vi "逐點分段offset改善、比較 2.vi"() -> ()   [LabVIEW 2017]
uses:
  <vilib>/Utility/miscctls.llb/LVPointDoubleTypeDef.ctl
panel:
  out "size(s)":i32
  out "Voltgae":dbl[](array[numeric])
  out "Voltage Position":cluster{"Speed":dbl[], "Position":dbl[]}(graph)
  out "element":T1
  in  "file path (use dialog)":path
  out "X  Position":dbl=1500.0
  out "max index(es)":i32=900
  out "Y max spped":dbl=50000.0
  out "NO OFFSET Graph":cluster{"Speed":dbl[], "Position":dbl[]}(graph)
  in  "OFFSET":dbl=0.6 format="%#_13g"
  out "OFFSET Graph":cluster{"Speed":dbl[], "Position":dbl[]}(graph)
  in  "X Position":T2={"Position 1"=100.0, "Position 2"=500.0, "Position 3"=1000.0, "Position 4"=1500.0, "Position 5"=2000.0, "Position 6"=2100.0} {"Position 6" step=100.0; "Position 5" step=100.0; "Position 4" step=100.0; "Position 3" step=100.0; "Position 2" step=100.0; "Position 1" step=100.0}
  in  "Y Speed":T3={"Speed 1"=1000.0, "Speed 2"=2000.0, "Speed 3"=3000.0, "Speed 4"=30000.0, "Speed 5"=50000.0, "Speed 6"=3000.0} {"Speed 6" step=100.0; "Speed 5" step=100.0; "Speed 4" step=100.0; "Speed 3" step=100.0; "Speed 2" step=100.0; "Speed 1" step=100.0}
  # "0.01mm"
  # "0.01mm"
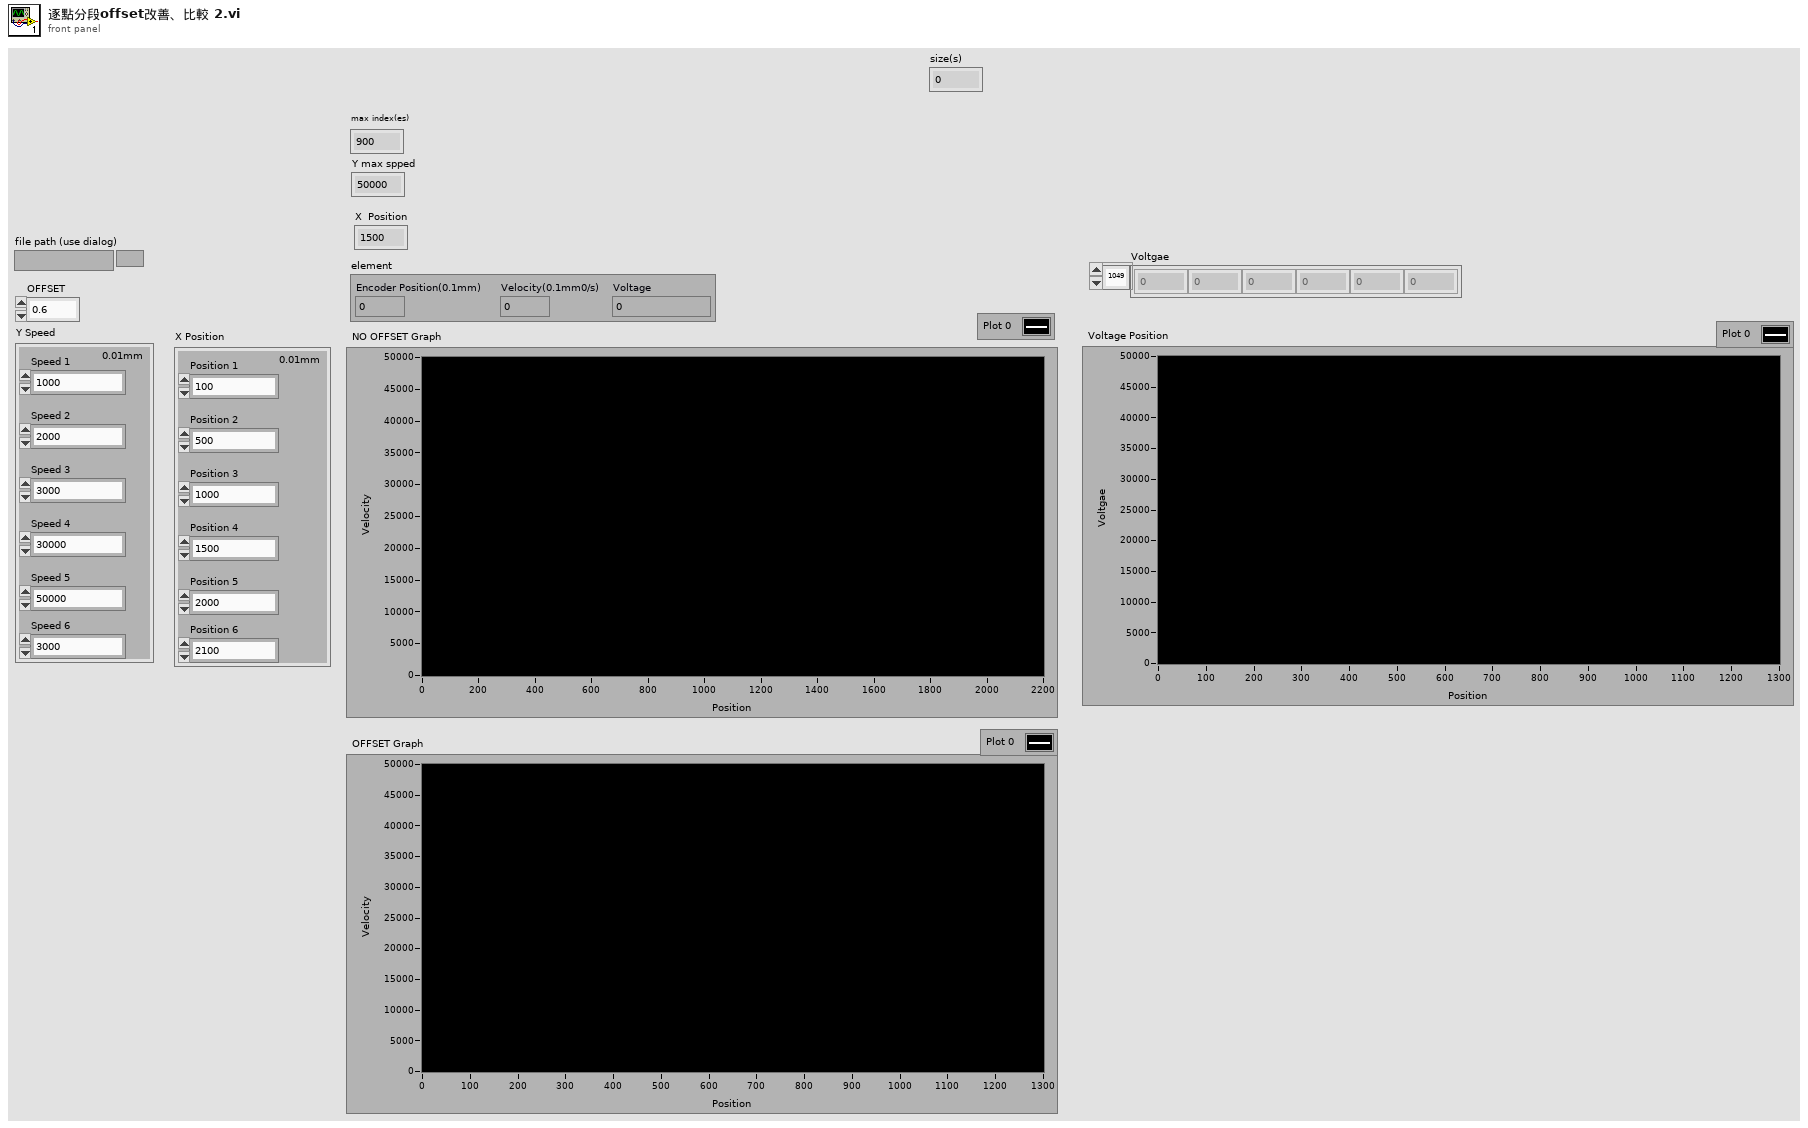
[diagram p1: front panel]
types:
  T1 = cluster{"Encoder Position(0.1mm)":dbl, "Velocity(0.1mm0/s)":dbl, "Voltage":dbl}
  T2 = cluster{"Position 1":dbl, "Position 2":dbl, "Position 3":dbl, "Position 4":dbl, "Position 5":dbl, "Position 6":dbl}
  T3 = cluster{"Speed 1":dbl, "Speed 2":dbl, "Speed 3":dbl, "Speed 4":dbl, "Speed 5":dbl, "Speed 6":dbl}
  T4 = typedef "LVPointDoubleTypeDef.ctl" = cluster{"X":dbl, "Y":dbl}
  T5 = cluster{"Real Periold(ms)":dbl[], "Encoder Position(0.1mm)":dbl[], "Velocity(0.1mm0/s)":dbl[], "Voltage":dbl[]}
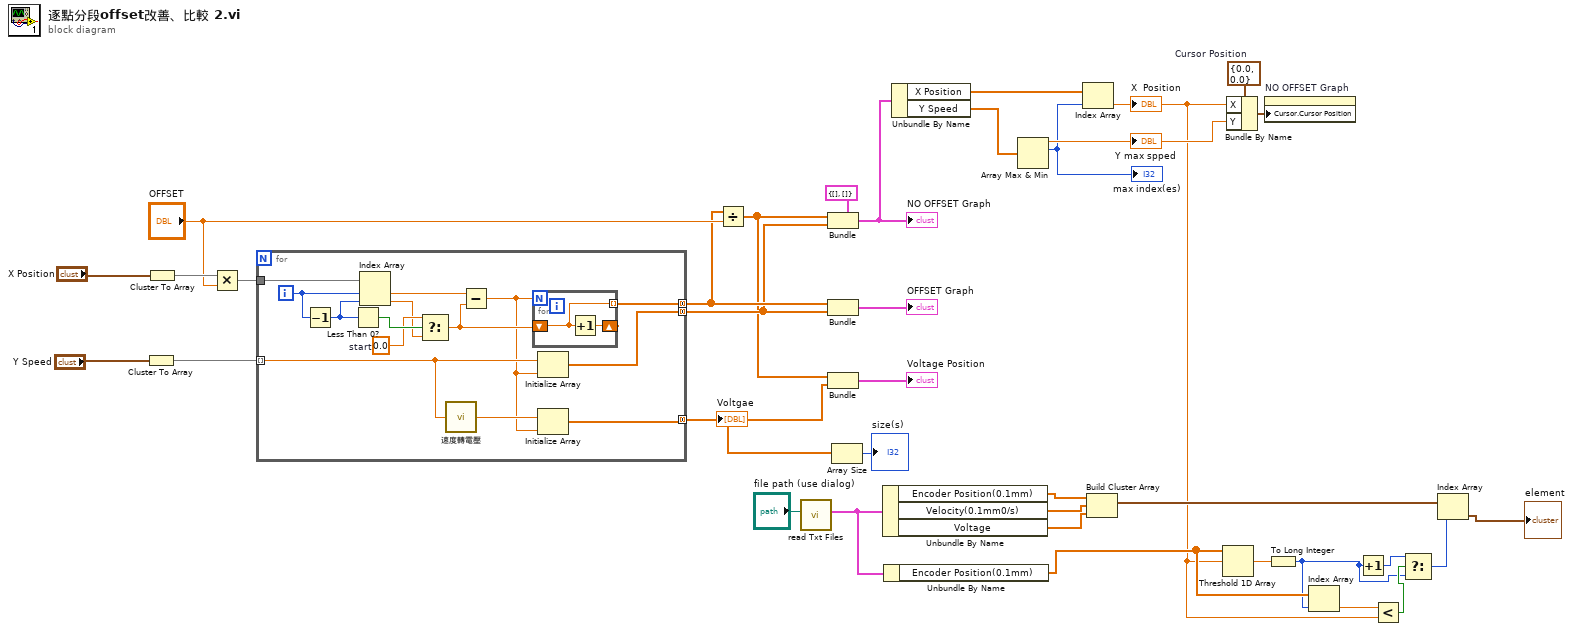
[diagram p0: block diagram]
diagram:
  w27 = T4 {"X"=0.0, "Y"=0.0}  # Cursor Position
  n1 = Cluster To Array(cluster="Y Speed") -> (array=w31:dbl[])
  n2 = Cluster To Array(cluster="X Position") -> (array=w32:dbl[])
  n3 = Multiply(x=w32, y="OFFSET") -> (x*y=w33:dbl[])
  n4 = for {
    tunnel: w33 -> [w50]
    tunnel: w31 -> [w40] mode=indexing
    tunnel: [w43] -> w29 mode=concatenating
    tunnel: [w44] -> w25 mode=concatenating
    tunnel: [w37] -> w2 mode=concatenating
    i -> [w49]
    w46 = 0.0  # start
    n5 = Decrement(x=w49) -> (x-1=w48:i32)
    n6 = Less Than 0?(x=w48) -> (x < 0?=w47:bool)
    n7 = Index Array(array=w50, index #1=w49, index #2=w48) -> (element #1=w41:dbl, element #2=w45:dbl)
    n8 = Select(t=w46, s=w47, f=w45) -> (s? t:f=w42:dbl)
    n9 = call "速度轉電壓.vi"("Speed (0.1mm/s)"=w40) -> ("Voltage\nOutput"=w39:dbl)
    n10 = Subtract(x=w41, y=w42) -> (x-y=w38:dbl)
    n11 = for {
      N: w38 -> [_]
      shift-right: [w52] -> _
      shift-left: w42 -> [w51]
      tunnel: [w51] -> w43 mode=indexing
      n12 = Increment(x=w51) -> (x+1=w52:dbl)
    }
    n13 = Initialize Array(w40, w38) -> (w44:dbl[])
    n14 = Initialize Array(w39, w38) -> (w37:dbl[])
  }
  "Voltgae" <- w2
  n15 = Divide(x=w29, y="OFFSET") -> (x/y=w4:dbl[])
  n16 = call "read Txt Files.vi"("file path (use dialog)"="file path (use dialog)") -> ("number"=w18:T5)  [unwired: 10 in]
  n17 = Bundle(cluster=cluster{"X Position":dbl[], "Y Speed":dbl[]} {"X Position"=[], "Y Speed"=[]}, "X Position"=w4, "Y Speed"=w25) -> (w22:cluster{"X Position":dbl[], "Y Speed":dbl[]})
  "NO OFFSET Graph" <- w22
  n18 = Bundle(w29, w25) -> (→"OFFSET Graph":cluster{dbl[], dbl[]})  [unwired: 1 in]
  n19 = Bundle(w4, w2) -> (→"Voltage Position":cluster{dbl[], dbl[]})  [unwired: 1 in]
  n20 = Array Size(array=w2) -> (size(s)=→"size(s)":i32)
  n21 = Unbundle By Name(w18) -> ("Encoder Position(0.1mm)"=w17:dbl[], "Velocity(0.1mm0/s)"=w16:dbl[], "Voltage"=w15:dbl[])
  n22 = Unbundle By Name(w18) -> ("Encoder Position(0.1mm)"=w11:dbl[])
  n23 = Unbundle By Name(w22) -> ("X Position"=w21:dbl[], "Y Speed"=w20:dbl[])
  n24 = Array Max & Min(array=w20) -> (max value=w26:dbl, max index (indices)=w24:i32)  [unwired: 2 out]
  "Y max spped" <- w26
  "max index(es)" <- w24
  n25 = Index Array(array=w21, index=w24) -> (element=w5:dbl)
  "X  Position" <- w5
  n26 = Build Cluster Array(w17, w16, w15) -> (w14:cluster{dbl, dbl, dbl}[])
  n27 = Threshold 1D Array(2:w5, 3:w11) -> (0:w13:dbl)  [unwired: 1 in]
  n28 = Bundle By Name(cluster=w27, "X"=w5, "Y"=w26) -> (w28:T4)
  n29 = property on="NO OFFSET Graph" class="XYGraph (strict)"("Cursor.Cursor Position"=w28) -> ()  [unwired: 2 in, 2 out]
  n30 = To Long Integer(number=w13) -> (32bit integer=w9:i32)
  n31 = Index Array(array=w11, index=w9) -> (element=w6:dbl)
  n32 = Increment(x=w9) -> (x+1=w8:i32)
  n33 = Less?(x=w6, y=w5) -> (x < y?=w10:bool)
  n34 = Select(t=w8, s=w10, f=w9) -> (s? t:f=w7:i32)
  n35 = Index Array(array=w14, index=w7) -> (element=→"element":cluster{dbl, dbl, dbl})
